vi "FPGAmain_5782_Fast_PID.vi"() -> ()   [LabVIEW 2013]
uses:
  FPGA/DataMode.ctl
  FPGA/Input_5782/5782_Fast_PID_states.ctl
  <vilib>/Platform/TimedLoop/XDataNode/timing_clust.ctl
  <vilib>/Platform/TimedLoop/XDataNode/nitl_modes.ctl
  <vilib>/Platform/TimedLoop/XDataNode/wakeup.ctl
  <vilib>/rvi/Emulation/niFpgaSctlEmulationGetInTimedLoop.vi
  <vilib>/rvi/Emulation/niFpgaEmulationReportErrorSimple.vi
  <vilib>/rvi/Emulation/niFpgaGetClockAttributes.vi
  <vilib>/rvi/eio/common/nirviEmuTemplateMethod_errors.vi
  <vilib>/rvi/Emulation/niFpgaCriticalErrorInLSC.vi
  <vilib>/rvi/FIFO/Fifo_Resource/nirvififoEmulationReadFpgaImpl.vi
  <vilib>/rvi/DataTransferAndStorage/Container/Common/niFpgaContainerGetUniqueNameForEmu.vi
  <vilib>/rvi/DataTransferAndStorage/Register/Emulation/niFpgaRegisterEmulationFpgaImpl.vi
  <instcachedir>/0/niFpgaRegisterEmulationFpgaImpl_DCF4BC0110594B98B44A971D60CEEC4D.lvgen/niFpgaRegisterEmulationFpgaImpl_DCF4BC0110594B98B44A971D60CEEC4D_010.vi
  <vilib>/rvi/interface/RandomDataEmulation/nirviRandomDataMultiElementFPGAFIFO.vi
  <instcachedir>/0/nirviRandomDataMultiElementFPGAFIFO_F2B80EDE0D7944A08478D8D26097D4DB.lvgen/nirviRandomDataMultiElementFPGAFIFO_F2B80EDE0D7944A08478D8D26097D4DB_000.vi
  <vilib>/rvi/interface/RandomDataEmulation/niFpgaRandomDataHandleErrors.vi
  <vilib>/rvi/interface/RandomDataEmulation/nirviRandomDataFPGAFIFO.vi
  <instcachedir>/0/niFpgaRegisterEmulationFpgaImpl_DCF4BC0110594B98B44A971D60CEEC4D.lvgen/niFpgaRegisterEmulationFpgaImpl_DCF4BC0110594B98B44A971D60CEEC4D_014.vi
  <vilib>/rvi/FIFO/Fifo_Resource/nirvififoEmulationWriteFpgaImpl.vi
  <instcachedir>/0/niFpgaRegisterEmulationFpgaImpl_DCF4BC0110594B98B44A971D60CEEC4D.lvgen/niFpgaRegisterEmulationFpgaImpl_DCF4BC0110594B98B44A971D60CEEC4D_016.vi
  <instcachedir>/0/niFpgaRegisterEmulationFpgaImpl_DCF4BC0110594B98B44A971D60CEEC4D.lvgen/niFpgaRegisterEmulationFpgaImpl_DCF4BC0110594B98B44A971D60CEEC4D_008.vi
  <instcachedir>/0/niFpgaRegisterEmulationFpgaImpl_DCF4BC0110594B98B44A971D60CEEC4D.lvgen/niFpgaRegisterEmulationFpgaImpl_DCF4BC0110594B98B44A971D60CEEC4D_009.vi
  <instcachedir>/0/niFpgaRegisterEmulationFpgaImpl_DCF4BC0110594B98B44A971D60CEEC4D.lvgen/niFpgaRegisterEmulationFpgaImpl_DCF4BC0110594B98B44A971D60CEEC4D_005.vi
  <instcachedir>/0/niFpgaRegisterEmulationFpgaImpl_DCF4BC0110594B98B44A971D60CEEC4D.lvgen/niFpgaRegisterEmulationFpgaImpl_DCF4BC0110594B98B44A971D60CEEC4D_006.vi
  <instcachedir>/0/niFpgaRegisterEmulationFpgaImpl_DCF4BC0110594B98B44A971D60CEEC4D.lvgen/niFpgaRegisterEmulationFpgaImpl_DCF4BC0110594B98B44A971D60CEEC4D_002.vi
  <instcachedir>/0/niFpgaRegisterEmulationFpgaImpl_DCF4BC0110594B98B44A971D60CEEC4D.lvgen/niFpgaRegisterEmulationFpgaImpl_DCF4BC0110594B98B44A971D60CEEC4D_003.vi
  <instcachedir>/0/niFpgaRegisterEmulationFpgaImpl_DCF4BC0110594B98B44A971D60CEEC4D.lvgen/niFpgaRegisterEmulationFpgaImpl_DCF4BC0110594B98B44A971D60CEEC4D_017.vi
  <instcachedir>/0/niFpgaRegisterEmulationFpgaImpl_DCF4BC0110594B98B44A971D60CEEC4D.lvgen/niFpgaRegisterEmulationFpgaImpl_DCF4BC0110594B98B44A971D60CEEC4D_019.vi
  <instcachedir>/0/niFpgaRegisterEmulationFpgaImpl_DCF4BC0110594B98B44A971D60CEEC4D.lvgen/niFpgaRegisterEmulationFpgaImpl_DCF4BC0110594B98B44A971D60CEEC4D_018.vi
  <instcachedir>/0/niFpgaRegisterEmulationFpgaImpl_DCF4BC0110594B98B44A971D60CEEC4D.lvgen/niFpgaRegisterEmulationFpgaImpl_DCF4BC0110594B98B44A971D60CEEC4D_004.vi
  <vilib>/Platform/TimedLoop/XDataNode/XDataNode.xnode
  <vilib>/eio/EIONode/EIONode.xnode
  <vilib>/rvi/DataTransferAndStorage/Container/XNode/niFpgaContainer.xnode
  <vilib>/rvi/FIFO/Fifo_Resource/nirvififoEmulationRead.vi
  <vilib>/rvi/DataTransferAndStorage/Register/Emulation/niFpgaRegisterEmulation.vi
  <vilib>/rvi/interface/RandomDataEmulation/nirviRandomDataFpgaMultiElementTemplate.vi
  <vilib>/rvi/interface/RandomDataEmulation/nirviRandomDataFpgaReadWriteTemplate.vi
  <vilib>/rvi/FIFO/Fifo_Resource/nirvififoEmulationWrite.vi
  <vilib>/Platform/TimedLoop/XDataNode/XDNodeRunTimeDep.lvlib
panel:
  in  "Full speed transfer":bool
  in  "IO Module\\AO Data Sync":bool=TRUE
  in  "IO Module\\SPI Write Data":u16
  out "IO Module\\SPI Read Data":u8
  in  "IO Module\\SPI Read":bool
  in  "IO Module\\SPI Write":bool
  in  "IO Module\\SPI Address":u16
  in  "IO Module\\SPI Device":u8
  out "IO Module\\SPI Idle":bool
  in  "AM phase":fxp<+,64,64>
  in  "delay phase":fxp<+,64,64>
  in  "User Command Commit":bool
  in  "User Command":u8
  out "User Command Idle":bool
  out "User Command Status":u8
  in  "User Data 0":u8
  in  "User Data 1":u8
  out "PLL Locked":bool
  out "User Error":bool
  out "Configured?":bool
  in  "Continuous":bool
  in  "5782 record length":u16=4000 caption="Samples Per Trigger" min=1 step=1
  in  "Trigger Acquisition":bool
  out "IO Module\\Trigger Input":bool
  in  "Downsample":fxp<+,8,8>=1.0
  in  "new coeffs":bool
  in  "FIR coeffs":fxp<+/-,18,18>[](array[numeric])
  in  "CIC Gain":fxp<+/-,32,1>=0.00390625 format="%#_32g"
  in  "Acquisition running":bool
  in  "Phase output":fxp<+,64,64>[](array[numeric])=[0.0, 0.0, 0.0, 0.0]
  in  "Simulated phase 5782":fxp<+,64,64>[](array[numeric])=[0.0, 0.0]
  in  "Mode":T1
  in  "Phase 5782":fxp<+,64,64>[](array[numeric])=[0.0, 0.0]
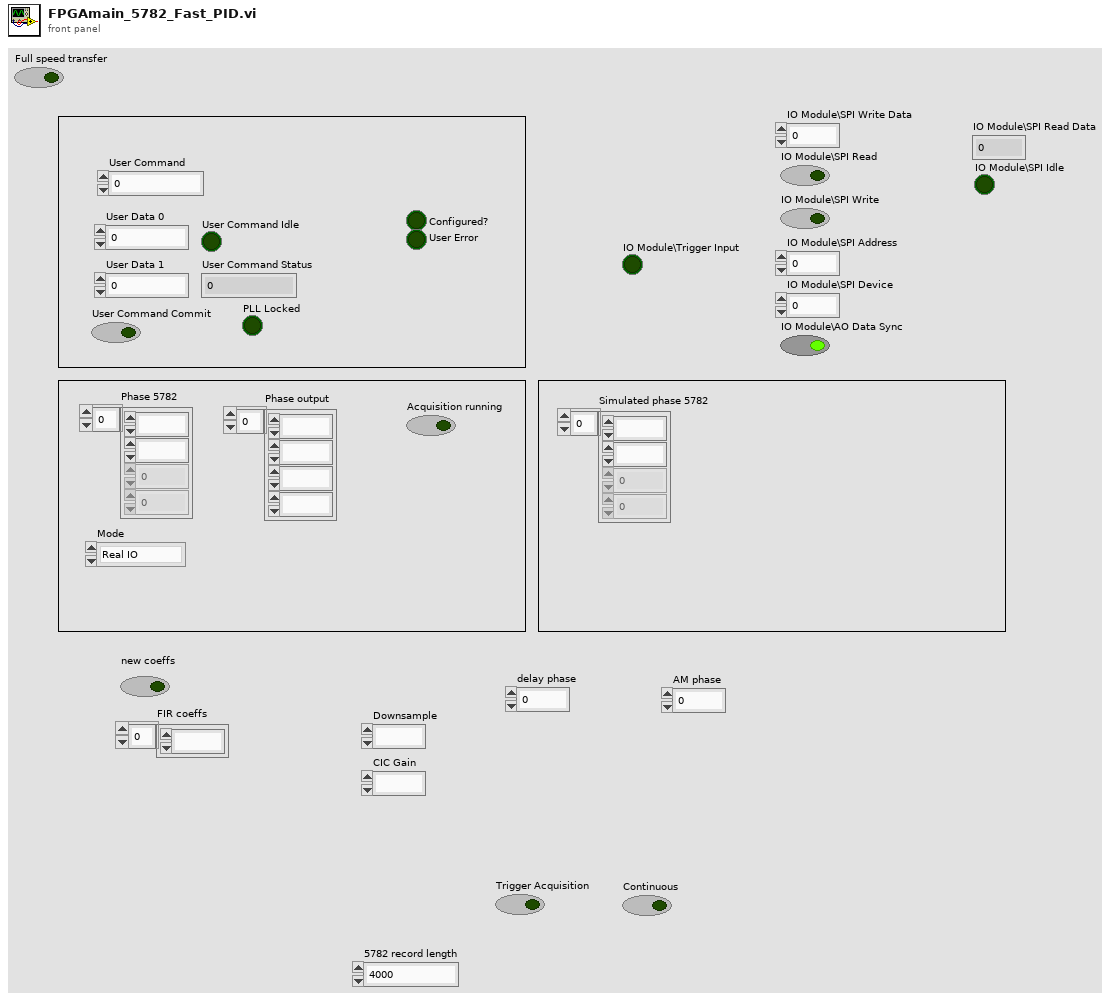
[diagram p1: front panel]
types:
  T1 = typedef "DataMode.ctl" = enum16{"Real IO", "Simulated"}
  T2 = typedef "5782_Fast_PID_states.ctl" = enum8{"Wait for trigger", "Acquisition", "Send record length", "Wait for output", "Quiet period"}
  T3 = typedef "XDNodeRunTimeDep.lvlib/timing_clust.ctl" = cluster{"Expected End [f-1]":u64, "Actual End [f-1]":u64, "Finished Late? [f-1]":bool, "Expected End [i-1]":u64, "Actual End [i-1]":u64, "Finished Late? [i-1]":bool, "Expected Start [i]":u64, "Actual Start [i]":u64, "Expected Start [f]":u64, "Actual Start [f]":u64, "Source Name":string, "Structure Name":string, "Period":i64, "Deadline":i64, "Offset":i64, "Start":i64, "Priority":i32, "Timeout":i32, "Mode":T4, "Wakeup Reason":T5, "Error":errorcluster, "Source Type":string, "Secondary Source Type":string, "Global End Time":u64, "Global Start Time":u64, "Frame Duration":u64, "Iteration Duration":u64, "Assigned CPU":i32, "I/O Scan Engine Mode":u32}
  T4 = typedef "XDNodeRunTimeDep.lvlib/nitl_modes.ctl" = enum32{"No Change", "Process missed periods, maintain original phase", "Discard missed periods, maintain original phase", "Process missed periods, ignore original phase", "Discard missed periods, ignore original phase"}
  T5 = typedef "XDNodeRunTimeDep.lvlib/wakeup.ctl" = enum32{"Normal", "Aborted", "Asynchronous wakeup", "Timing source error", "Timed loop error", "Timeout"}
  T6 = typedef "I16 array size 2.ctl" = i16[]
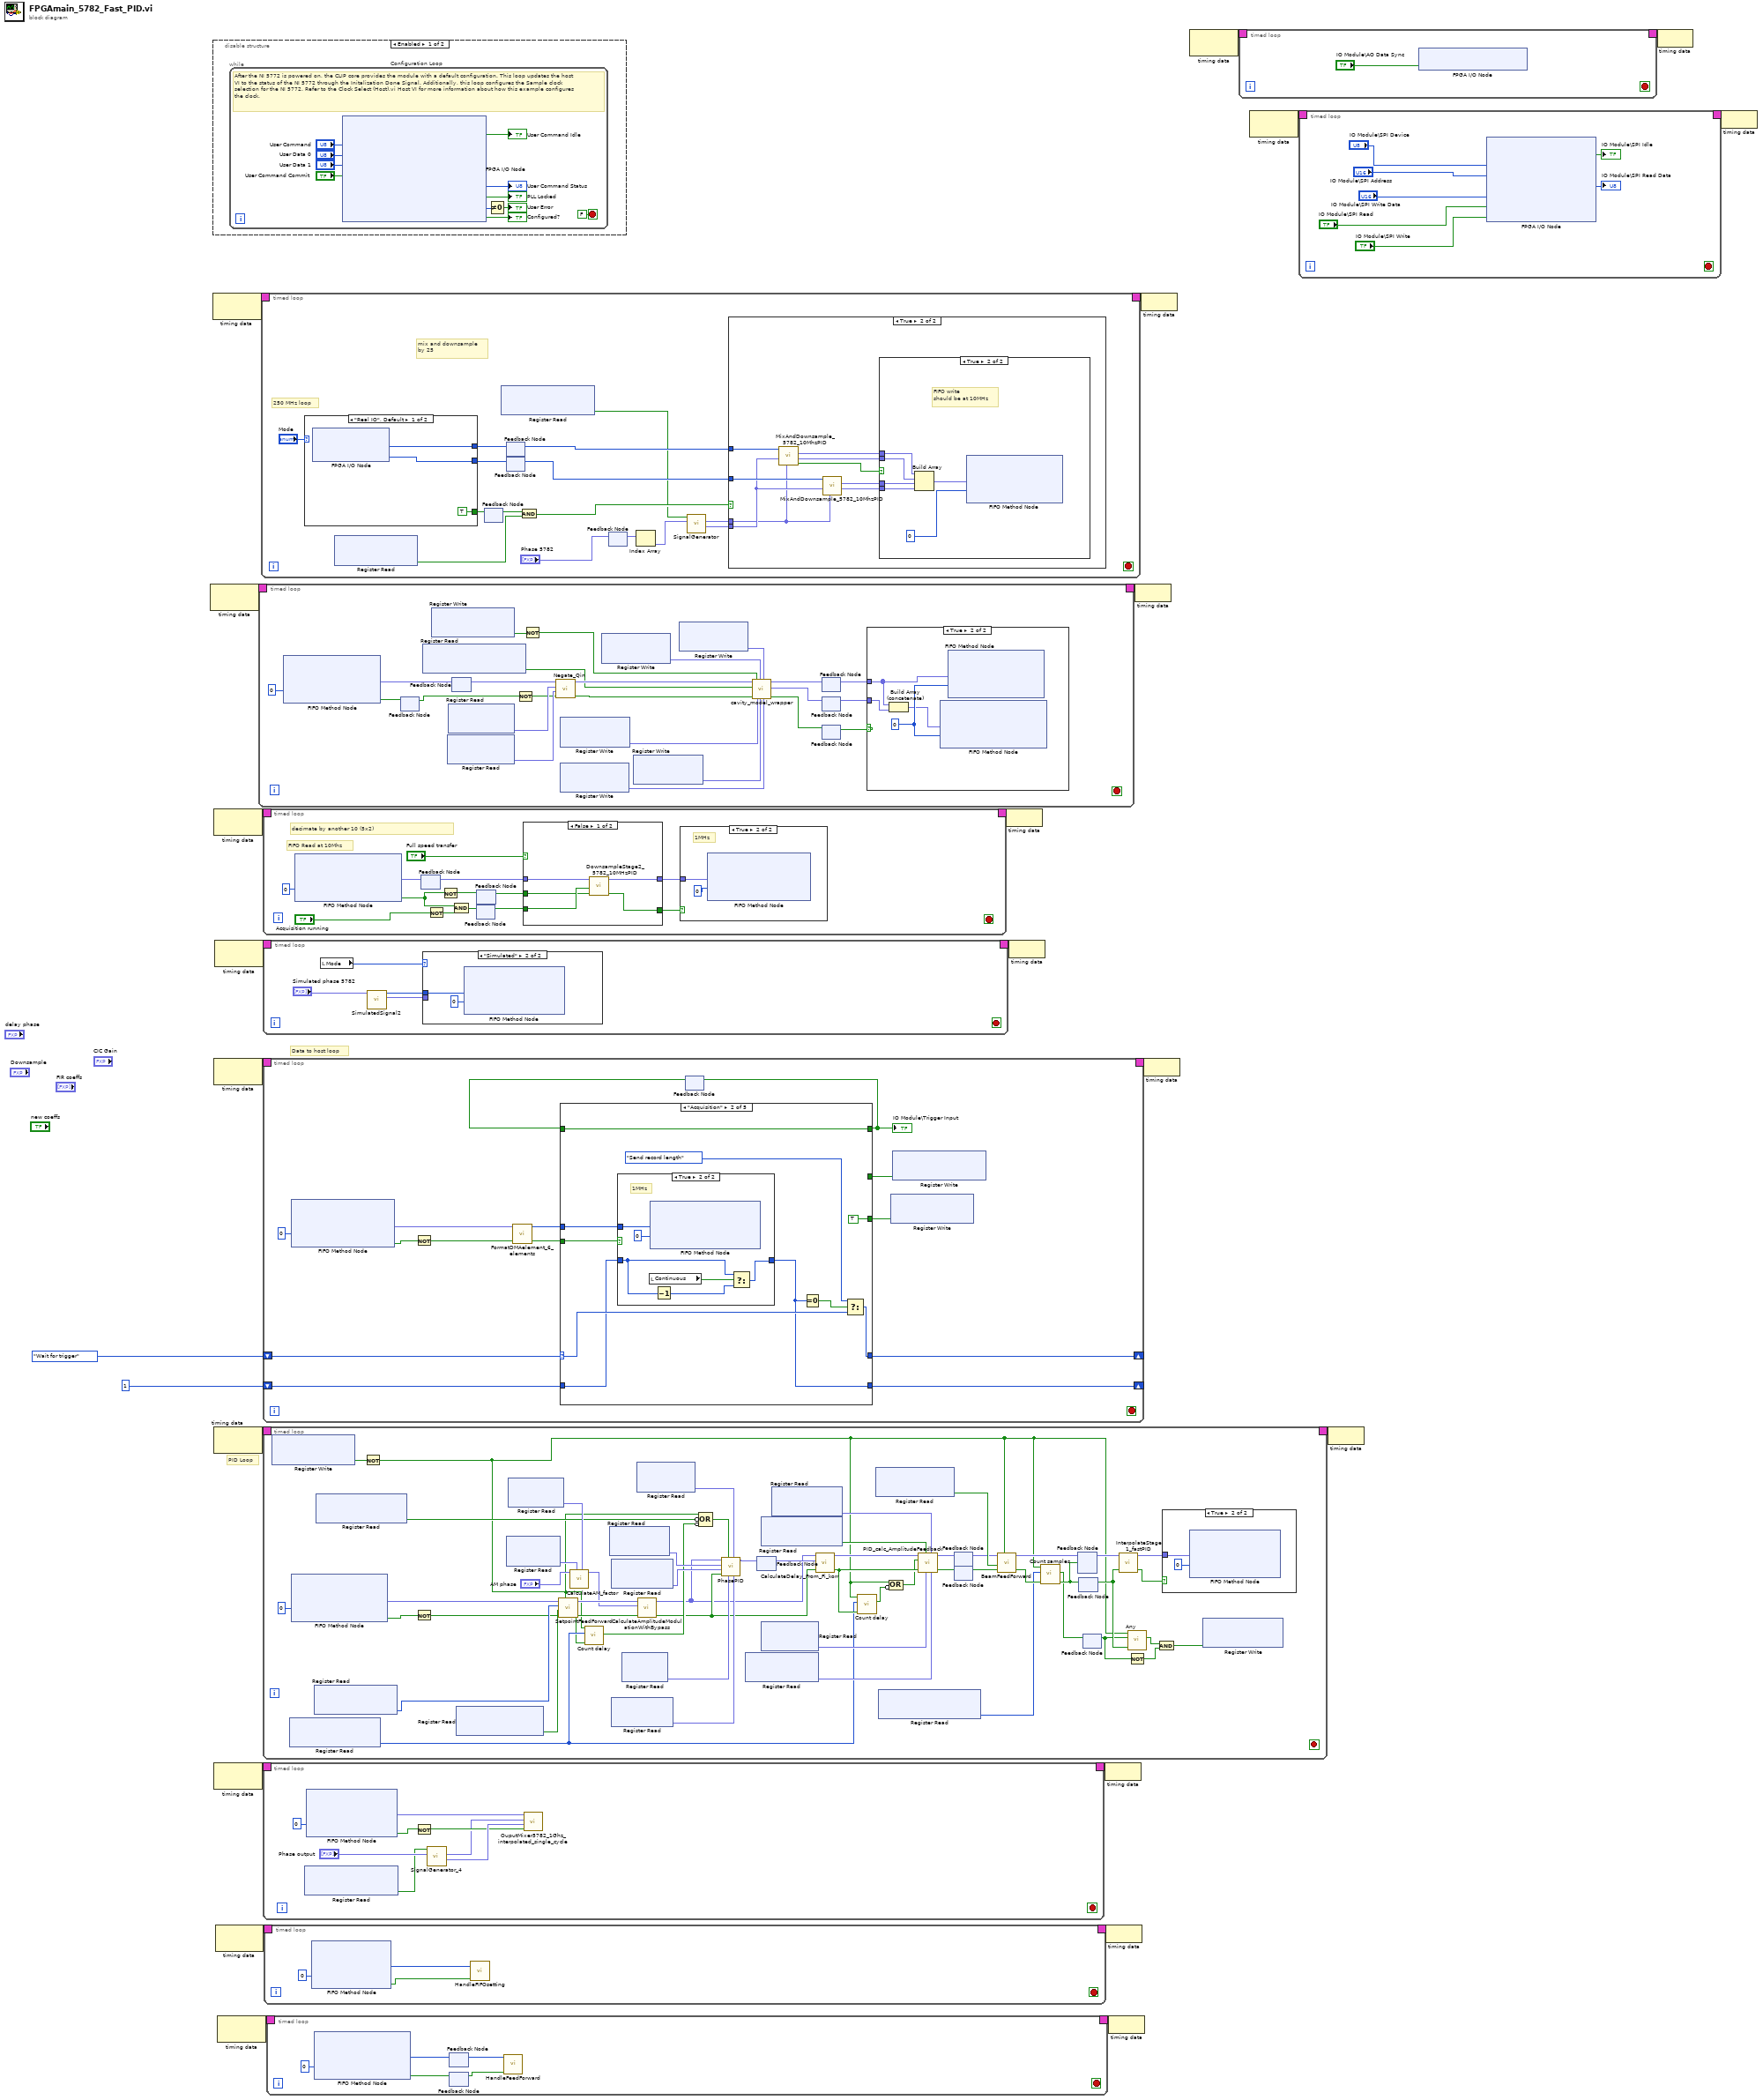
[diagram p0: block diagram]
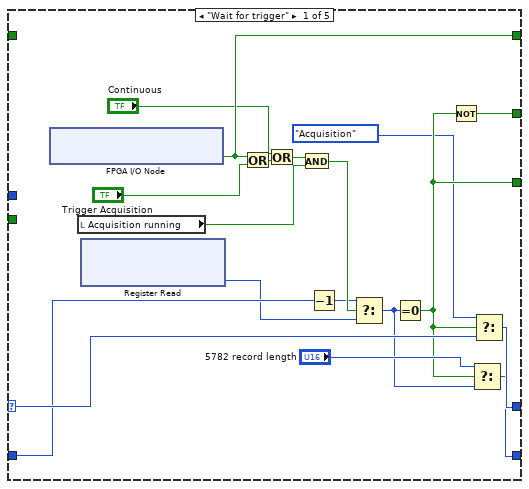
[diagram p3: hidden frame]
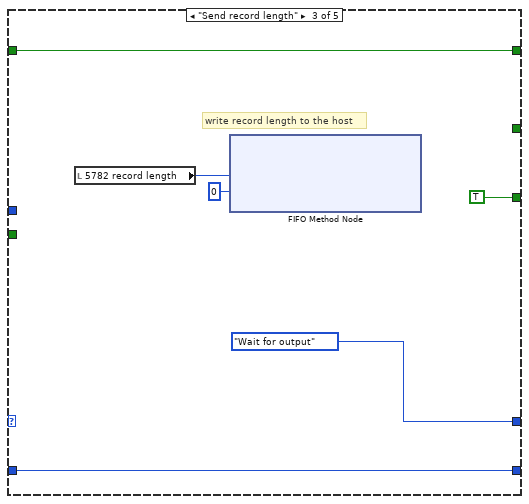
[diagram p5: hidden frame]
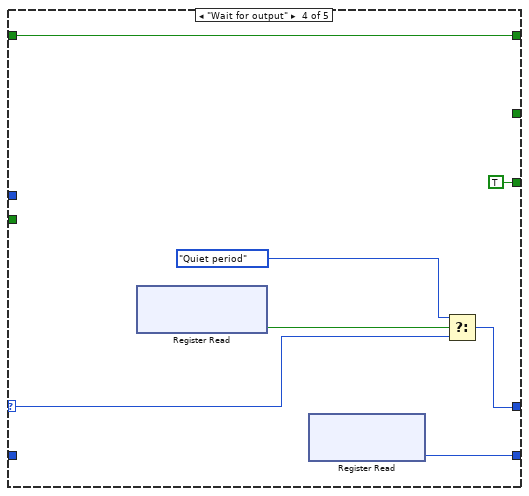
[diagram p6: hidden frame]
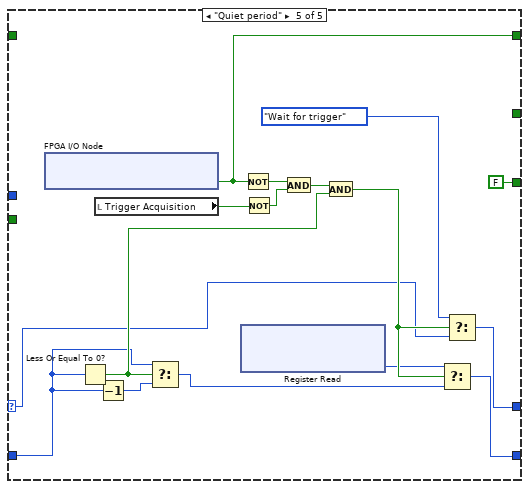
[diagram p7: hidden frame]
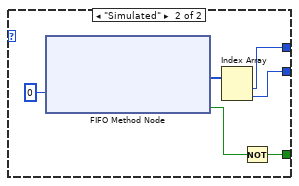
[diagram p14: hidden frame]
diagram:
  # "PID Loop"
  # "Data to host loop"
  n1 = node-c288() -> (w2:T3)  [unwired: 1 in]
  n2 = node-c288() -> (w22:T3)  [unwired: 1 in]
  n3 = disable-structure shown="Enabled" {
    frame Enabled {
      n4 = while "Configuration Loop" {
        stop <- FALSE stop-if-true
        # "After the NI 5772 is powered on, the CLIP core provides the module with a default configuration. This loop updates the host VI to the status of the NI 5772 through the Initalization Done Signal. Additionally, this loop configures the Sample clock selection for the NI 5772. Refer to the Clock Select (Host).vi Host VI for more information about how this example configures the clock."
        n5 = xnode "FPGA I/O Node"("IO Module\\User Command"="User Command", "IO Module\\User Data 0"="User Data 0", "IO Module\\User Data 1"="User Data 1", "IO Module\\User Command Commit"="User Command Commit") -> ("IO Module\\User Command Idle"=→"User Command Idle":bool, "IO Module\\User Command Status"=→"User Command Status":u8, "IO Module\\PLL Locked"=→"PLL Locked":bool, "IO Module\\User Error"=w30:u8, "IO Module\\Initialization Done"=→"Configured?":bool)  [unwired: 9 in, 9 out]
        n6 = Not Equal To 0?(x=w30) -> (x != 0?=→"User Error":bool)
      }
    }
    frame Disabled {
    }
  }
  n7 = node-c288() -> (w9:T3)  [unwired: 1 in]
  n8 = node-c288() -> (w7:T3)  [unwired: 1 in]
  n9 = node-c288() -> (w11:T3)  [unwired: 1 in]
  n10 = node-c288() -> (w17:T3)  [unwired: 1 in]
  n11 = node-c288() -> (w24:T3)  [unwired: 1 in]
  n12 = node-c288() -> (w19:T3)  [unwired: 1 in]
  n13 = node-c288() -> (w4:T3)  [unwired: 1 in]
  n14 = timed-loop {
    timing: w2 -> [_]
    timing-out: [_] -> w1
    stop <- _ stop-if-true
    n15 = xnode ("FIFO Method Node")("Timeout"=0) -> ("Element"=w45:fxp<+/-,16,14>[], "Timed Out?"=w44:bool)  [unwired: 1 in, 1 out]
    n16 = feedback #1() -> (w42:bool)  [unwired: 1 in]
    n17 = feedback-in #1(w44) -> ()
    n18 = xnode ("Register Read")() -> ("Data"=w53:bool)  [unwired: 1 in, 1 out]
    n19 = xnode ("Register Write")() -> ("Data"=w52:bool)  [unwired: 1 in, 1 out]
    n20 = xnode ("Register Read")() -> ("Data"=w58:fxp<+/-,16,14>)  [unwired: 1 in, 1 out]
    n21 = xnode ("Register Read")() -> ("Data"=w59:fxp<+/-,16,14>)  [unwired: 1 in, 1 out]
    n22 = feedback #2() -> (w43:fxp<+/-,16,14>[])  [unwired: 1 in]
    n23 = feedback-in #2(w45) -> ()
    n24 = Not(x=w42) -> (.not. x?=w57:bool)
    n25 = Not(x=w52) -> (.not. x?=w54:bool)
    n26 = call "Negate_Qin.vi"("valid in"=w57, "DC offset chan 1"=w58, "DC offset chan 0"=w59, "Data in"=w43) -> ("valid out"=w55:bool, "Data out"=w56:fxp<+/-,16,14>[])  [unwired: 6 in]
    n27 = xnode ("Register Write")() -> ("Data"=w38:fxp<+/-,32,-40>)  [unwired: 1 in, 1 out]
    n28 = xnode ("Register Write")() -> ("Data"=w36:fxp<+/-,32,3>)  [unwired: 1 in, 1 out]
    n29 = xnode ("Register Write")() -> ("Data"=w39:fxp<+/-,32,3>)  [unwired: 1 in, 1 out]
    n30 = xnode ("Register Write")() -> ("Data"=w37:fxp<+/-,32,2>)  [unwired: 1 in, 1 out]
    n31 = xnode ("Register Write")() -> ("Data"=w40:fxp<+/-,32,3>)  [unwired: 1 in, 1 out]
    n32 = call "cavity_model_wrapper.vi"("Data in"=w56, "enabled"=w53, "input valid"=w55, "reset"=w54, "C3"=w36, "C1"=w39, "C4"=w37, "C2"=w40, "C5"=w38) -> ("Data out"=w51:fxp<+/-,16,14>[], "Ai1 out"=w47:fxp<+/-,16,14>[], "output valid"=w49:bool)  [unwired: 8 in]
    n33 = feedback #3() -> (w50:fxp<+/-,16,14>[])  [unwired: 1 in]
    n34 = feedback-in #3(w51) -> ()
    n35 = feedback #4() -> (w46:fxp<+/-,16,14>[])  [unwired: 1 in]
    n36 = feedback-in #4(w47) -> ()
    n37 = feedback #5() -> (w48:bool)  [unwired: 1 in]
    n38 = feedback-in #5(w49) -> ()
    n39 = case shown="True" w48 {
      tunnel: w50 -> [_ w62]
      tunnel: w46 -> [_ w61]
      frame False {
      }
      frame True {
        w63 = 0 ("Timeout")
        n40 = Build Array (concatenate)(w62, w61) -> (w60:fxp<+/-,16,14>[])
        n41 = xnode ("FIFO Method Node")("Element"=w60, "Timeout"=w63) -> ()  [unwired: 1 in, 2 out]
        n42 = xnode ("FIFO Method Node")("Element"=w62, "Timeout"=w63) -> ()  [unwired: 1 in, 2 out]
      }
    }
  }
  n43 = timed-loop {
    timing: w22 -> [_]
    timing-out: [_] -> w21
    stop <- _ stop-if-true
    # "mix and downsample\nby 25"
    # "250 MHz loop"
    n44 = case shown="\"Real IO\", Default" "Mode" {
      tunnel: [w98 w101] -> w79
      tunnel: [w97 w102] -> w77
      tunnel: [TRUE w99] -> w75
      frame "Real IO", Default {
        n45 = xnode "FPGA I/O Node"() -> ("IO Module\\AI 0"=w98:i16, "IO Module\\AI 1"=w97:i16)  [unwired: 2 in, 2 out]
      }
      frame "Simulated" {
        n46 = xnode ("FIFO Method Node")("Timeout"=0) -> ("Element"=w103:i16[], "Timed Out?"=w100:bool)  [unwired: 1 in, 1 out]
        n47 = Index Array(array=w103) -> (element #1=w101:i16, element #2=w102:i16)  [unwired: 2 in]
        n48 = Not(x=w100) -> (.not. x?=w99:bool)
      }
    }
    n49 = xnode ("Register Read")() -> ("Data"=w73:bool)  [unwired: 1 in, 1 out]
    n50 = feedback #6() -> (w74:bool)  [unwired: 1 in]
    n51 = feedback-in #6(w75) -> ()
    n52 = xnode ("Register Read")() -> ("Data"=w66:bool)  [unwired: 1 in, 1 out]
    n53 = feedback #7() -> (w78:i16)  [unwired: 1 in]
    n54 = feedback-in #7(w79) -> ()
    n55 = feedback #8() -> (w76:i16)  [unwired: 1 in]
    n56 = feedback-in #8(w77) -> ()
    n57 = And(x=w74, y=w73) -> (x .and. y?=w67:bool)
    n58 = feedback #9() -> (w72:fxp<+,64,64>[])  [unwired: 1 in]
    n59 = feedback-in #9("Phase 5782") -> ()
    n60 = Index Array(array=w72) -> (element=w71:fxp<+,64,64>)  [unwired: 1 in]
    n61 = call "SignalGenerator.vi"("phase"=w71, "Reset"=w66) -> ("Cos"=w69:fxp<+/-,16,0>, "Sin"=w68:fxp<+/-,16,0>)  [unwired: 7 in, 1 out]
    n62 = case shown="True" w67 {
      tunnel: w78 -> [_ w89]
      tunnel: w76 -> [_ w88]
      tunnel: w69 -> [_ w82]
      tunnel: w68 -> [_ w81]
      frame False {
      }
      frame True {
        n63 = call "MixAndDownsample_5782_10MhzPID.vi"("sin0"=w81, "cos0"=w82, "signal 0"=w89) -> ("data valid"=w85:bool, "Q out"=w86:fxp<+/-,16,14>, "I out"=w87:fxp<+/-,16,14>)  [unwired: 6 in]
        n64 = call "MixAndDownsample_5782_10MhzPID.vi"("sin0"=w81, "cos0"=w82, "signal 0"=w88) -> ("Q out"=w83:fxp<+/-,16,14>, "I out"=w84:fxp<+/-,16,14>)  [unwired: 6 in, 1 out]
        n65 = case shown="True" w85 {
          tunnel: w86 -> [_ w95]
          tunnel: w87 -> [_ w94]
          tunnel: w84 -> [_ w93]
          tunnel: w83 -> [_ w92]
          frame False {
          }
          frame True {
            # "FIFO write\nshould be at 10MHz"
            n66 = Build Array(w94, w95, w93, w92) -> (w91:fxp<+/-,16,14>[])
            n67 = xnode ("FIFO Method Node")("Element"=w91, "Timeout"=0) -> ()  [unwired: 1 in, 2 out]
          }
        }
      }
    }
  }
  n68 = timed-loop {
    timing: w9 -> [_]
    timing-out: [_] -> w8
    stop <- _ stop-if-true
    # "FIFO Read at 10Mhz"
    # "decimate by another 10 (5x2)"
    n69 = xnode ("FIFO Method Node")("Timeout"=0) -> ("Element"=w115:fxp<+/-,16,14>[], "Timed Out?"=w116:bool)  [unwired: 1 in, 1 out]
    n70 = feedback #10() -> (w114:fxp<+/-,16,14>[])  [unwired: 1 in]
    n71 = feedback-in #10(w115) -> ()
    n72 = Not(x="Acquisition running") -> (.not. x?=w108:bool)
    n73 = Not(x=w116) -> (.not. x?=w110:bool)
    n74 = And(x=w116, y=w108) -> (x .and. y?=w112:bool)
    n75 = feedback #11() -> (w111:bool)  [unwired: 1 in]
    n76 = feedback-in #11(w112) -> ()
    n77 = feedback #12() -> (w109:bool)  [unwired: 1 in]
    n78 = feedback-in #12(w110) -> ()
    n79 = case shown="False" "Full speed transfer" {
      tunnel: [w124 w126] -> w118
      tunnel: [w123 w125] -> w117
      tunnel: w114 -> [w122 w126]
      tunnel: w111 -> [w121 _]
      tunnel: w109 -> [w120 w125]
      frame False {
        n80 = call "DownsampleStage2_5782_10MHzPID.vi"("valid in"=w120, "reset"=w121, "Data in"=w122) -> ("valid out"=w123:bool, "data out"=w124:fxp<+/-,16,14>[])  [unwired: 7 in]
      }
      frame True {
      }
    }
    n81 = case shown="True" w117 {
      tunnel: w118 -> [_ w127]
      frame False {
      }
      frame True {
        # "1MHz"
        n82 = xnode ("FIFO Method Node")("Element"=w127, "Timeout"=0) -> ()  [unwired: 1 in, 2 out]
      }
    }
  }
  n83 = timed-loop {
    timing: w7 -> [_]
    timing-out: [_] -> w6
    shift-right: [w142] -> _
    shift-left: 5782_Fast_PID_states."Wait for trigger" ("5782 states") -> [w144]
    shift-right: [w141] -> _
    shift-left: u16 1 ("trigger samples") -> [w143]
    stop <- _ stop-if-true
    n84 = xnode ("FIFO Method Node")("Timeout"=0) -> ("Element"=w132:fxp<+/-,16,14>[], "Timed Out?"=w139:bool)  [unwired: 1 in, 1 out]
    n85 = Not(x=w139) -> (.not. x?=w131:bool)
    n86 = call "FormatDMAelement_6_elements.vi"("valid in"=w131, "Data in"=w132) -> ("valid out"=w135:bool, "Values"=w134:u64[])  [unwired: 8 in]
    n87 = feedback #13() -> (w137:bool)  [unwired: 1 in]
    n88 = case shown="\"Acquisition\"" w144 {
      selector: w144 -> [w162 w172 _ w190 w194]
      tunnel: w143 -> [w152 w169 w180 _ w195]
      tunnel: [w161 w171 5782_Fast_PID_states."Wait for output" ("5782 states") w192 w207] -> w142
      tunnel: [w160 w166 w180 w188 w208] -> w141
      tunnel: w134 -> [_ w167 _ _ _]
      tunnel: w135 -> [_ w168 _ _ _]
      tunnel: [w147 TRUE TRUE ("5782 triggered") TRUE ("5782 triggered") FALSE ("5782 triggered")] -> w138
      tunnel: [w155 w165 w182 w186 w200] -> w136
      tunnel: w137 -> [_ w165 w182 w186 _]
      tunnel: [w146 _ _ _ _] -> w133
      frame "Wait for trigger" {
        n89 = xnode "FPGA I/O Node"() -> ("IO Module\\Trigger Input"=w155:bool)  [unwired: 1 in, 1 out]
        n90 = local read "Acquisition running"() -> (w156:bool)
        n91 = xnode ("Register Read")() -> ("Data"=w148:u16)  [unwired: 1 in, 1 out]
        n92 = Or(x=w155, y="Trigger Acquisition") -> (x .or. y?=w151:bool)
        n93 = Or(x="Continuous", y=w151) -> (x .or. y?=w149:bool)
        n94 = And(x=w149, y=w156) -> (x .and. y?=w157:bool)
        n95 = Decrement(x=w152) -> (x-1=w153:u16)
        n96 = Select(t=w153, s=w157, f=w148) -> (s? t:f=w154:u16)
        n97 = Equal To 0?(x=w154) -> (x = 0?=w147:bool)
        n98 = Not(x=w147) -> (.not. x?=w146:bool)
        n99 = Select(t="5782 record length", s=w147, f=w154) -> (s? t:f=w160:u16)
        n100 = Select(t=5782_Fast_PID_states."Acquisition" ("5782 states"), s=w147, f=w162) -> (s? t:f=w161:T2)
      }
      frame "Acquisition" {
        n101 = case shown="True" w168 {
          tunnel: w167 -> [_ w179]
          tunnel: [w173 w176] -> w166
          tunnel: w169 -> [w173 w174]
          frame False {
          }
          frame True {
            # "1MHz"
            n102 = local read "Continuous"() -> (w177:bool)
            n103 = xnode ("FIFO Method Node")("Element"=w179, "Timeout"=0) -> ()  [unwired: 1 in, 2 out]
            n104 = Decrement(x=w174) -> (x-1=w175:u16)
            n105 = Select(t=w174, s=w177, f=w175) -> (s? t:f=w176:u16)
          }
        }
        n106 = Equal To 0?(x=w166) -> (x = 0?=w170:bool)
        n107 = Select(t=5782_Fast_PID_states."Send record length" ("5782 states"), s=w170, f=w172) -> (s? t:f=w171:T2)
      }
      frame "Send record length" {
        # "write record length to the host"
        n108 = local read "5782 record length"() -> (w184:u16)
        n109 = xnode ("FIFO Method Node")("Element"=w184, "Timeout"=0) -> ()  [unwired: 1 in, 2 out]
      }
      frame "Wait for output" {
        n110 = xnode ("Register Read")() -> ("Data"=w187:bool)  [unwired: 1 in, 1 out]
        n111 = xnode ("Register Read")() -> ("Data"=w188:u16)  [unwired: 1 in, 1 out]
        n112 = Select(t=5782_Fast_PID_states."Quiet period" ("5782 states"), s=w187, f=w190) -> (s? t:f=w192:T2)
      }
      frame "Quiet period" {
        n113 = xnode "FPGA I/O Node"() -> ("IO Module\\Trigger Input"=w200:bool)  [unwired: 1 in, 1 out]
        n114 = Less Or Equal To 0?(x=w195) -> (x <= 0?=w198:bool)
        n115 = local read "Trigger Acquisition"() -> (w205:bool)
        n116 = Decrement(x=w195) -> (x-1=w199:u16)
        n117 = Select(t=w195, s=w198, f=w199) -> (s? t:f=w197:u16)
        n118 = xnode ("Register Read")() -> ("Data"=w196:u16)  [unwired: 1 in, 1 out]
        n119 = Not(x=w200) -> (.not. x?=w204:bool)
        n120 = Not(x=w205) -> (.not. x?=w203:bool)
        n121 = And(x=w204, y=w203) -> (x .and. y?=w202:bool)
        n122 = And(x=w202, y=w198) -> (x .and. y?=w206:bool)
        n123 = Select(t=w196, s=w206, f=w197) -> (s? t:f=w208:u16)
        n124 = Select(t=5782_Fast_PID_states."Wait for trigger" ("5782 states"), s=w206, f=w194) -> (s? t:f=w207:T2)
      }
    }
    "IO Module\\Trigger Input" <- w136
    n125 = feedback-in #13(w136) -> ()
    n126 = xnode ("Register Write")("Data"=w138) -> ()  [unwired: 1 in, 1 out]
    n127 = xnode ("Register Write")("Data"=w133) -> ()  [unwired: 1 in, 1 out]
  }
  n128 = timed-loop {
    timing: w11 -> [_]
    timing-out: [_] -> w10
    stop <- _ stop-if-true
    n129 = xnode ("Register Write")() -> ("Data"=w250:bool)  [unwired: 1 in, 1 out]
    n130 = xnode ("Register Read")() -> ("Data"=w223:u32)  [unwired: 1 in, 1 out]
    n131 = xnode ("FIFO Method Node")("Timeout"=0) -> ("Element"=w212:fxp<+/-,16,14>[], "Timed Out?"=w262:bool)  [unwired: 1 in, 1 out]
    n132 = xnode ("Register Read")() -> ("Data"=w214:u32)  [unwired: 1 in, 1 out]
    n133 = xnode ("Register Read")() -> ("Data"=w229:bool)  [unwired: 1 in, 1 out]
    n134 = Not(x=w250) -> (.not. x?=w213:bool)
    n135 = Not(x=w262) -> (.not. x?=w211:bool)
    n136 = xnode ("Register Read")() -> ("Data"=w249:bool)  [unwired: 1 in, 1 out]
    n137 = xnode ("Register Read")() -> ("Data"=w255:fxp<+/-,16,2>)  [unwired: 1 in, 1 out]
    n138 = xnode ("Register Read")() -> ("Data"=w254:fxp<+/-,16,2>)  [unwired: 1 in, 1 out]
    n139 = call "SetpointFeedForward.vi"("Reset"=w213, "input valid"=w211, "setpoint enabled"=w249, "Samples to skip"=w214, "Data in"=w212) -> ("output valid"=w220:bool, "Data out"=w221:fxp<+/-,16,14>[])  [unwired: 5 in]
    n140 = call "CalculateAM_factor.vi"("b_am"=w254, "a_am"=w255, "AM phase"="AM phase") -> ("AM_factor"=w215:fxp<+/-,16,2>)  [unwired: 7 in, 1 out]
    n141 = call "Count delay.vi"("input valid"=w220, "Count to skip"=w223, "Reset"=w213) -> ("count done?"=w228:bool)  [unwired: 7 in, 1 out]
    n142 = xnode ("Register Read")() -> ("Data"=w258:fxp<+/-,32,4>)  [unwired: 1 in, 1 out]
    n143 = xnode ("Register Read")() -> ("Data"=w259:fxp<+/-,32,4>)  [unwired: 1 in, 1 out]
    n144 = xnode ("Register Read")() -> ("Data"=w260:fxp<+/-,32,4>)  [unwired: 1 in, 1 out]
    n145 = xnode ("Register Read")() -> ("Data"=w261:fxp<+/-,32,4>)  [unwired: 1 in, 1 out]
    n146 = xnode ("Register Read")() -> ("Data"=w257:fxp<+/-,32,4>)  [unwired: 1 in, 1 out]
    n147 = call "CalculateAmplitudeModulationWithBypass.vi"("input valid"=w220, "AM_factor"=w215, "Data in"=w221) -> ("output valid"=w219:bool, "Data out"=w218:fxp<+/-,16,14>[])  [unwired: 7 in]
    n148 = Compound Arithmetic op=OR(w213, invert w229, invert w228) -> (w227:bool)
    n149 = call "PhasePID.vi"("Kd/Tau"=w260, "Ki*Tau"=w257, "Kp"=w261, "Reset"=w227, "input valid"=w219, "Fi_delta"=w259, "Fi_start"=w258, "Data in"=w218) -> ("Fi_korr PID"=w256:fxp<+/-,32,4>)  [unwired: 1 in, 2 out]
    n150 = xnode ("Register Read")() -> ("Data"=w240:fxp<+/-,32,6>)  [unwired: 1 in, 1 out]
    n151 = feedback-in #14(w256) -> ()
    n152 = feedback #14() -> (w248:fxp<+/-,32,4>)  [unwired: 1 in]
    n153 = xnode ("Register Read")() -> ("Data"=w241:fxp<+/-,32,6>)  [unwired: 1 in, 1 out]
    n154 = xnode ("Register Read")() -> ("Data"=w244:bool)  [unwired: 1 in, 1 out]
    n155 = xnode ("Register Read")() -> ("Data"=w243:fxp<+/-,32,6>)  [unwired: 1 in, 1 out]
    n156 = call "CalculateDelay_From_Fi_korr.vi"("input valid"=w219, "fi_korr"=w248, "Data in"=w218) -> ("output valid"=w226:bool, "Data out"=w242:fxp<+/-,16,14>[])  [unwired: 7 in]
    n157 = call "Count delay.vi"("input valid"=w226, "Count to skip"=w223, "Reset"=w213) -> ("count done?"=w225:bool)  [unwired: 7 in, 1 out]
    n158 = xnode ("Register Read")() -> ("Data"=w239:bool)  [unwired: 1 in, 1 out]
    n159 = xnode ("Register Read")() -> ("Data"=w222:u32)  [unwired: 1 in, 1 out]
    n160 = Compound Arithmetic op=OR(w213, invert w225) -> (w224:bool)
    n161 = call "PID_calc_AmplitudeFeedback.vi"("Kd/Tau"=w240, "Ki*Tau"=w243, "Kp"=w241, "Enabled"=w244, "input valid"=w226, "Reset"=w224, "Data in"=w242) -> ("output valid"=w245:bool, "data out"=w246:fxp<+/-,16,14>[])  [unwired: 1 in, 2 out]
    n162 = feedback #15() -> (w216:fxp<+/-,16,14>[])  [unwired: 1 in]
    n163 = feedback-in #15(w246) -> ()
    n164 = feedback #16() -> (w217:bool)  [unwired: 1 in]
    n165 = feedback-in #16(w245) -> ()
    n166 = call "BeamFeedForward.vi"("Reset"=w213, "input valid"=w217, "beam enabled"=w239, "Data in"=w216) -> ("output valid"=w237:bool, "Data out"=w247:fxp<+/-,16,14>[])  [unwired: 6 in]
    n167 = call "Count samples.vi"("input valid"=w237, "number to count"=w222, "Reset"=w213) -> ("output valid"=w238:bool, "counting"=w235:bool)  [unwired: 7 in]
    n168 = feedback #17() -> (w236:fxp<+/-,16,14>[])  [unwired: 1 in]
    n169 = feedback-in #17(w247, w238) -> ()
    n170 = feedback #18() -> (w234:bool)  [unwired: 1 in]
    n171 = feedback-in #18(w238) -> ()
    n172 = feedback #19() -> (w233:bool)  [unwired: 1 in]
    n173 = feedback-in #19(w235) -> ()
    n174 = call "InterpolateStage1_fastPID.vi"("valid in"=w234, "Data in"=w236) -> ("valid out"=w251:bool, "Data out"=w252:fxp<+/-,16,14>[])  [unwired: 8 in]
    n175 = call "Any.vi"("input valid"=w234, "Value"=w233, "Reset"=w213) -> ("Any?"=w232:bool)  [unwired: 7 in, 1 out]
    n176 = Not(x=w233) -> (.not. x?=w231:bool)
    n177 = And(x=w232, y=w231) -> (x .and. y?=w230:bool)
    n178 = case shown="True" w251 {
      tunnel: w252 -> [_ w265]
      frame False {
      }
      frame True {
        n179 = xnode ("FIFO Method Node")("Element"=w265, "Timeout"=0) -> ()  [unwired: 1 in, 2 out]
      }
    }
    n180 = xnode ("Register Write")("Data"=w230) -> ()  [unwired: 1 in, 1 out]
  }
  n181 = timed-loop {
    timing: w17 -> [_]
    timing-out: [_] -> w16
    stop <- _ stop-if-true
    n182 = xnode ("Register Read")() -> ("Data"=w268:bool)  [unwired: 1 in, 1 out]
    n183 = xnode ("FIFO Method Node")("Timeout"=0) -> ("Element"=w271:fxp<+/-,16,14>[], "Timed Out?"=w274:bool)  [unwired: 1 in, 1 out]
    n184 = Not(x=w274) -> (.not. x?=w270:bool)
    n185 = call "SignalGenerator_4.vi"("Phase"="Phase output", "reset"=w268) -> ("Sine out"=w272:fxp<+/-,16,0>[], "Cosine out"=w269:fxp<+/-,16,0>[])  [unwired: 8 in]
    n186 = call "OuputMixer5782_1Ghz_interpolated_single_cycle.vi"("input valid"=w270, "Sine in"=w272, "Cosine in"=w269, "Data"=w271) -> ()  [unwired: 7 in, 1 out]
  }
  n187 = timed-loop {
    timing: w24 -> [_]
    timing-out: [_] -> w23
    stop <- _ stop-if-true
    n188 = local read "Mode"() -> (w281:T1)
    n189 = call "SimulatedSignal2.vi"("Phase"="Simulated phase 5782") -> ("dummy do not use"=w278:fxp<+/-,16,0>[], "output"=w280:T6)  [unwired: 9 in]
    n190 = case shown="\"Simulated\"" w281 {
      tunnel: w280 -> [_ w282]
      tunnel: w278 -> [_ _]
      frame "Real IO", Default {
      }
      frame "Simulated" {
        n191 = xnode ("FIFO Method Node")("Element"=w282, "Timeout"=0) -> ()  [unwired: 1 in, 2 out]
      }
    }
  }
  n192 = timed-loop {
    timing: w19 -> [_]
    timing-out: [_] -> w18
    stop <- _ stop-if-true
    n193 = xnode ("FIFO Method Node")("Timeout"=0) -> ("Element"=w287:u64, "Timed Out?"=w286:bool)  [unwired: 1 in, 1 out]
    n194 = call "HandleFIFOsetting.vi"("timed out"=w286, "Value"=w287) -> ()  [unwired: 10 in]
  }
  n195 = timed-loop {
    timing: w4 -> [_]
    timing-out: [_] -> w3
    stop <- _ stop-if-true
    n196 = xnode ("FIFO Method Node")("Timeout"=0) -> ("Element"=w294:u64, "Timed Out?"=w292:bool)  [unwired: 1 in, 1 out]
    n197 = feedback #20() -> (w293:u64)  [unwired: 1 in]
    n198 = feedback-in #20(w294) -> ()
    n199 = feedback #21() -> (w291:bool)  [unwired: 1 in]
    n200 = feedback-in #21(w292) -> ()
    n201 = call "HandleFeedForward.vi"("timed out"=w291, "Value"=w293) -> ()  [unwired: 10 in]
  }
  n202 = node-c288(w8) -> ()
  n203 = node-c288(w23) -> ()
  n204 = node-c288(w16) -> ()
  n205 = node-c288(w18) -> ()
  n206 = node-c288(w3) -> ()
  n207 = node-c288(w1) -> ()
  n208 = node-c288(w21) -> ()
  n209 = node-c288(w6) -> ()
  n210 = node-c288() -> (w13:T3)  [unwired: 1 in]
  n211 = timed-loop {
    timing: w13 -> [_]
    timing-out: [_] -> w12
    stop <- _ stop-if-true
    n212 = xnode "FPGA I/O Node"("IO Module\\AO Data Sync"="IO Module\\AO Data Sync") -> ()  [unwired: 1 in, 1 out]
  }
  n213 = node-c288() -> (w15:T3)  [unwired: 1 in]
  n214 = timed-loop {
    timing: w15 -> [_]
    timing-out: [_] -> w14
    stop <- _ stop-if-true
    n215 = xnode "FPGA I/O Node"("IO Module\\SPI Device"="IO Module\\SPI Device", "IO Module\\SPI Address"="IO Module\\SPI Address", "IO Module\\SPI Write Data"="IO Module\\SPI Write Data", "IO Module\\SPI Read"="IO Module\\SPI Read", "IO Module\\SPI Write"="IO Module\\SPI Write") -> ("IO Module\\SPI Idle"=→"IO Module\\SPI Idle":bool, "IO Module\\SPI Read Data"=→"IO Module\\SPI Read Data":u8)  [unwired: 7 in, 7 out]
  }
  n216 = node-c288(w10) -> ()
  n217 = node-c288(w12) -> ()
  n218 = node-c288(w14) -> ()
